vi "Pose_New_TRRO.vi"(9 "ROTATION":T3={"VALUE"=0.0, "COS"=1.0, "SIN"=0.0}, 11 "TRANSLATION":T2) -> (3 "outPOSE":T1={"TRANSLATION"={"X"=0.0, "Y"=0.0}, "ROTATION"={"VALUE"=0.0, "COS"=1.0, "SIN"=0.0}})   [LabVIEW 2019, in "Trajectory_Library.lvlib"]
doc: "Constructs a pose with the specified translation and rotation.\n\nParameters:\n - translation - The translational component of the pose.\n - rotation - The rotational component of the pose.\n\nReturn:\n - POSE - Pose data structure"
uses:
  Trajectory_Library.lvlib
  TRANSLATION2D.ctl
  ROTATION2D.ctl
  POSE2D.ctl
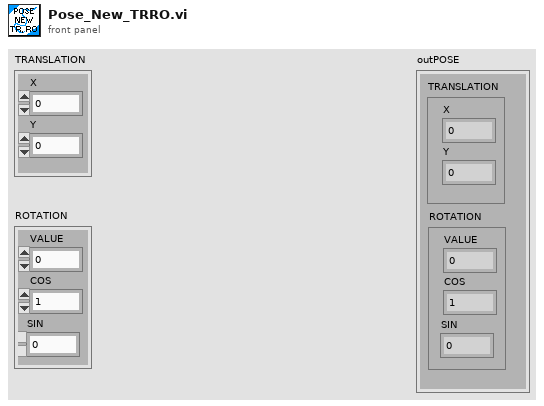
[diagram p1: front panel]
types:
  T1 = typedef "Trajectory_Library.lvlib/POSE2D.ctl" = cluster{"TRANSLATION":T2, "ROTATION":T3}
  T2 = typedef "Trajectory_Library.lvlib/TRANSLATION2D.ctl" = cluster{"X":dbl, "Y":dbl}
  T3 = typedef "Trajectory_Library.lvlib/ROTATION2D.ctl" = cluster{"VALUE":dbl, "COS":dbl, "SIN":dbl}
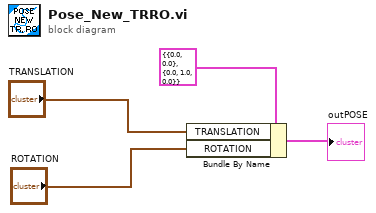
[diagram p0: block diagram]
diagram:
  n1 = Bundle By Name(cluster=T1 {"TRANSLATION"={"X"=0.0, "Y"=0.0}, "ROTATION"={"VALUE"=0.0, "COS"=1.0, "SIN"=0.0}} ("POSE"), "TRANSLATION"="TRANSLATION", "ROTATION"="ROTATION") -> (→"outPOSE":T1)
